vi "Custom Assertion Failure Message.vi"() -> ()   [LabVIEW 2017, in "Assertion.Tests.lvlib" / "Assert No Error.lvlib"]
uses:
  Assert No Error.lvlib
  <vilib>/Utility/error.llb/Error Cluster From Error Code.vi
  <vilib>/ErrorRing/Error Ring.xnode
  Assertion/Assertion.lvlib
panel:
  out "error out":errorcluster
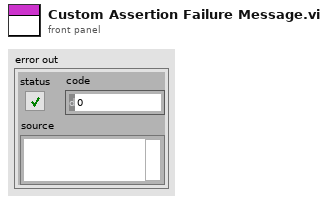
[diagram p1: front panel]
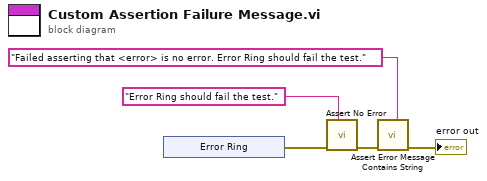
[diagram p0: block diagram]
diagram:
  n1 = xnode "Error Ring"() -> ("error out"=w5:errorcluster)
  n2 = call "Assert No Error.vi"("Message (\"\")"="Error Ring should fail the test." ("Message (\"\")"), "error in (no error)"=w5) -> ("error out"=w4:errorcluster)  [unwired: 9 in]
  n3 = call "Assert Error Message Contains String.vi"("Expected"="Failed asserting that <error> is no error. Error Ring should fail the test." ("Needle"), "error in (no error)"=w4) -> ("error out"=→"error out":errorcluster)  [unwired: 9 in]
